vi "Write Data - Byte (Scalar).vi"(5 "Data Block #":u16, 6 "Start Address":T1, 7 "Memory Area":T2 items=["P Area"=128, "I Area"=129, "O Area"=130, "M Area"=131, "DB Area"=132, "Counter"=40, "Timer"=41], 8 "error in (no error)":errorcluster, 10 "Value":u8, 11 "S7 in":refnum<class "S7NetCom.lvclass">) -> (0 "error out":errorcluster, 3 "S7 out":refnum<class "S7NetCom.lvclass">)   [LabVIEW 2014, in "S7NetCom.lvclass"]
doc: "Writes a single BYTE (U8) value to the PLC. \n_____\nCopyright (c) 2019 Hampel Software Engineering (HSE), released under BSD license. More info can be found on https://dokuwiki.hampel-soft.com/code/hse/s7netcom. Original code published by Marc Christenson, Sisu Devices."
uses:
  S7NetCom.lvclass
  Controls/S7_Memory_Area.ctl
  Controls/S7_Start_Address.ctl
  Controls/S7_Variable_Type.ctl
  S7NetCom.lvclass/S7NetCom.ctl
  SubVIs/TPKT/TPKT - Write Packet.vi
  SubVIs/COTP/COTP - Add Header.vi
  SubVIs/COTP/COTP - Validate Response Header.vi
  SubVIs/S7COMM/S7COMM - Parse Response - Decode Data Item.vi
  SubVIs/S7COMM/S7COMM - Evaluate Response Item Return Code.vi
  SubVIs/S7COMM/S7COMM - Parse Response - Evaluate Header.vi
  SubVIs/S7COMM/S7COMM - Parse Response - Evaluate Params.vi
  SubVIs/TPKT/TPKT - Add Header.vi
  Accessors/Get Timeout.vi
  Accessors/Get TCP Ref.vi
  Accessors/Set TCP Ref.vi
  SubVIs/COTP/COTP - Header for Data Transfer--constant.vi
  SubVIs/COTP/COTP - Response Header Mismatch--error.vi
  SubVIs/S7COMM/S7COMM - Parse Response - Decode Read Item - Split Data Array.vi
  SubVIs/S7COMM/S7COMM - Get Size Factor from Transport Data Type.vi
  SubVIs/S7COMM/S7COMM - Response Item Return Code-error.vi
  SubVIs/S7COMM/S7COMM - Header - Protocol ID--constant.vi
  Accessors/Get Sequence Number.vi
  SubVIs/S7COMM/S7COMM - Evaluate Protocol Header.vi
  SubVIs/S7COMM/S7COMM - Evaluate Message Type.vi
  SubVIs/S7COMM/S7COMM - Evaluate Sequence Number.vi
  SubVIs/S7COMM/S7COMM - Evaluate Response Error Code.vi
  SubVIs/TPKT/TPKT - Header Bytes 1 and 2--constant.vi
  SubVIs/S7COMM/S7COMM - Response Protocol Header Mismatch-error.vi
  SubVIs/S7COMM/S7COMM - Response Message Type Mismatch-error.vi
  SubVIs/S7COMM/S7COMM - Response Sequence Number Mismatch-error.vi
  SubVIs/S7COMM/S7COMM - Response Error Code-error.vi
  SubVIs/TPKT/TPKT - Read Packet.vi
panel:
  # "More info on https://dokuwiki.hampel-soft.com/code/hse/s7netcom\n\nCopyright (c) 2019, HAMPEL SOFTWARE ENGINEERING (HSE)\nOriginal code developed by Marc Christenson, Sisu Devices\nAll rights reserved.\n\nRedistribution and use in source and binary forms, with or without\nmodification, are permitted provided that the following conditions are met:\n\n1. Redistributions of source code must retain the above copyright\n   notice, this list of conditions and the following disclaimer.\n\n2. Redistributions in binary form must reproduce the above copyright\n   notice, this list of conditions and the following disclaimer in the\n   documentation and/or other materials provided with the distribution.\n\n3. All advertising materials mentioning features or use of this software\n   must display the following acknowledgement:\n   This product includes software developed by HAMPEL SOFTWARE ENGINEERING.\n\n4. Neither the name of HAMPEL SOFTWARE ENGINEERING nor the\n   names of its contributors may be used to endorse or promote products\n   derived from this software without specific prior written permission.\n\nTHIS SOFTWARE IS PROVIDED BY HAMPEL SOFTWARE ENGINEERING ''AS IS'' AND ANY\nEXPRESS OR IMPLIED WARRANTIES, INCLUDING, BUT NOT LIMITED TO, THE IMPLIED\nWARRANTIES OF MERCHANTABILITY AND FITNESS FOR A PARTICULAR PURPOSE ARE\nDISCLAIMED. IN NO EVENT SHALL HAMPEL SOFTWARE ENGINEERING BE LIABLE FOR ANY\nDIRECT, INDIRECT, INCIDENTAL, SPECIAL, EXEMPLARY, OR CONSEQUENTIAL DAMAGES\n(INCLUDING, BUT NOT LIMITED TO, PROCUREMENT OF SUBSTITUTE GOODS OR SERVICES;\nLOSS OF USE, DATA, OR PROFITS; OR BUSINESS INTERRUPTION) HOWEVER CAUSED AND\nON ANY THEORY OF LIABILITY, WHETHER IN CONTRACT, STRICT LIABILITY, OR TORT\n(INCLUDING NEGLIGENCE OR OTHERWISE) ARISING IN ANY WAY OUT OF THE USE OF THIS\nSOFTWARE, EVEN IF ADVISED OF THE POSSIBILITY OF SUCH DAMAGE."
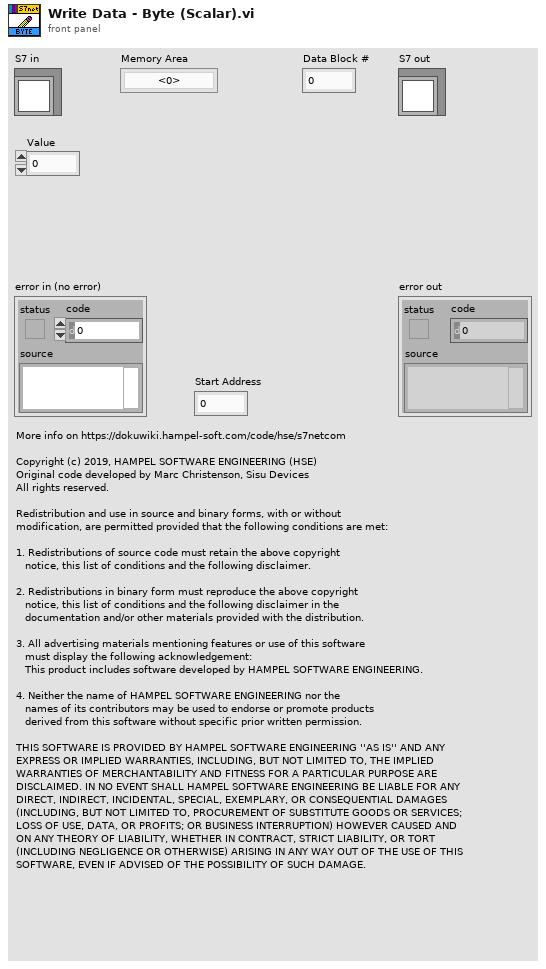
[diagram p1: front panel]
types:
  T1 = typedef "S7NetCom.lvclass/S7_Start_Address.ctl" = u16
  T2 = typedef "S7NetCom.lvclass/S7_Memory_Area.ctl" = u8
  T3 = typedef "S7NetCom.lvclass/S7_Variable_Type.ctl" = enum8{"---", "BIT", "BYTE", "CHAR", "WORD", "INT", "DWORD", "DINT", "REAL"}
  T4 = typedef "S7NetCom.lvclass/S7NetCom_HexByteArray.ctl" = T5[]
  T5 = typedef "S7NetCom.lvclass/S7NetCom_HexByte.ctl" = u8
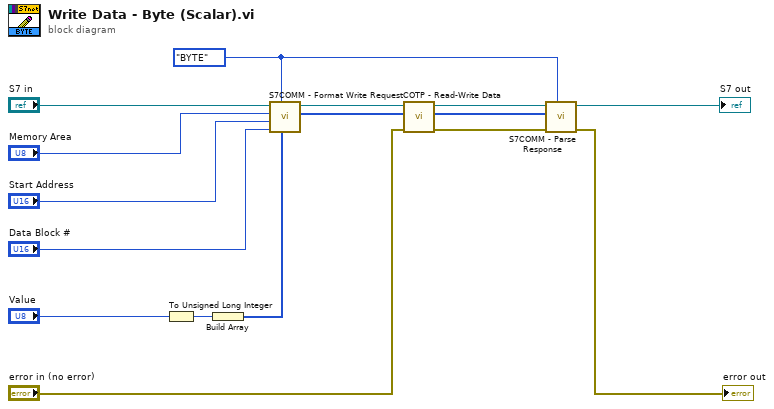
[diagram p0: block diagram]
diagram:
  w7 = S7_Variable_Type."BYTE" ("Variable Type")
  n1 = To Unsigned Long Integer(number="Value") -> (unsigned 32bit integer=w1:u32)
  n2 = Build Array(w1) -> (w2:u32[])
  n3 = call "S7COMM - Format Write Request.vi"("Data"=w2, "Variable Type"=w7, "Data Block #"="Data Block #", "Start Address"="Start Address", "Memory Area"="Memory Area", "S7"="S7 in") -> ("S7 PDU Data"=w14:T4, "S7 out"=w11:refnum<class "S7NetCom.lvclass">)  [unwired: 4 in]
  n4 = call "COTP - Read-Write Data.vi"("error in (no error)"="error in (no error)", "S7 PDU in"=w14, "S7 in"=w11) -> ("error out"=w5:errorcluster, "S7 PDU out"=w6:T4, "S7 out"=w15:refnum<class "S7NetCom.lvclass">)  [unwired: 6 in]
  n5 = call "S7COMM - Parse Response.vi"("Variable Type"=w7, "error in (no error)"=w5, "S7 PDU Data"=w6, "S7"=w15) -> ("error out"=→"error out":errorcluster, "S7 out"=→"S7 out":refnum<class "S7NetCom.lvclass">)  [unwired: 4 in, 2 out]
